vi "Start Measurements.vi"(6 "Reply to":refnum<class "Result Reply Msg.lvclass">, 7 "Objects enqueuers":refnum<class "Message Enqueuer.lvclass">[](array[class]), 8 "error in (no error)":errorcluster, 10 "Objects":string[](array[string]), 11 "Monitor Controller in":refnum<class "Monitor Controller.lvclass">) -> (0 "error out":errorcluster, 3 "Monitor Controller out":refnum<class "Monitor Controller.lvclass">)   [LabVIEW 2016, in "Monitor Controller.lvclass"]
uses:
  Monitor Controller.lvclass
  C:/github/LabActor/Worker/Worker.lvclass
  C:/github/LabActor/Controllers/Process Controller/Process Controller.lvclass
  Template Module Messages/Result Reply Msg/Result Reply Msg.lvclass
  <vilib>/ActorFramework/Message Enqueuer/Message Enqueuer.lvclass
  Worker/Worker.lvclass/Worker.ctl
  Monitor Controller.lvclass/Monitor Controller.ctl
  Process Controller/Process Controller.lvclass/Process Controller.ctl
  Worker/Write Cycle period.vi
  Process Controller/Write Repeat times.vi
  Process Controller/Write Timestamp data points.vi
  Template Module/Read State.vi
  Read Monitor controller configuration.vi
  Process Controller/Process Controller.lvclass
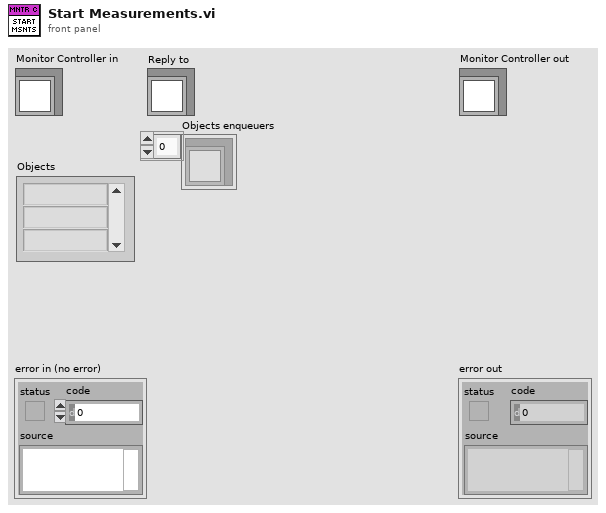
[diagram p1: front panel]
types:
  T1 = typedef "Worker State.ctl" = enum16{"Idle", "Starting", "Working", "Stopping"}
  T2 = typedef "Monitor Controller Configuration.ctl" = cluster{"Update period":dbl, "Repeat times":i32, "Open plot":bool, "File defragment period":dbl, "Timestamp data points":bool, "Re-plot rate limit":dbl}
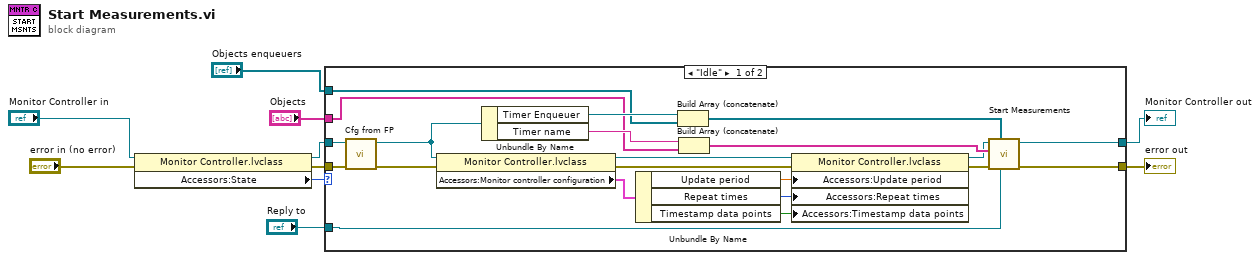
[diagram p0: block diagram]
diagram:
  n1 = property class="Monitor Controller.lvclass"(reference="Monitor Controller in", error in="error in (no error)") -> (reference out=w5:refnum<class "Monitor Controller.lvclass">, error out=w3:errorcluster, "Accessors:State"=w1:T1)
  n2 = case shown="\"Idle\"" w1 {
    tunnel: "Reply to" -> [w31 _]
    tunnel: "Objects enqueuers" -> [w29 _]
    tunnel: "Objects" -> [w27 _]
    tunnel: [w23 w32] -> w6
    tunnel: w5 -> [w15 w33]
    tunnel: w3 -> [w14 w32]
    tunnel: [w24 w33] -> w2
    frame "Idle" {
      n3 = call-dynamic "Cfg from FP.vi"("error in (no error)"=w14, "Measure Object in"=w15) -> ("error out"=w13:errorcluster, "Measure Object out"=w12:refnum<class "Monitor Controller.lvclass">)  [unwired: 8 in]
      n4 = property class="Monitor Controller.lvclass"(reference=w12, error in=w13) -> (reference out=w21:refnum<class "Monitor Controller.lvclass">, error out=w17:errorcluster, "Accessors:Monitor controller configuration"=w20:T2)
      n5 = Unbundle By Name(w12) -> ("Timer Enqueuer"=w30:refnum<class "Message Enqueuer.lvclass">, "Timer name"=w28:string)
      n6 = Unbundle By Name(w20) -> ("Update period"=w19:dbl, "Repeat times"=w16:i32, "Timestamp data points"=w11:bool)
      n7 = Build Array (concatenate)(w30, w29) -> (w26:refnum<class "Message Enqueuer.lvclass">[])
      n8 = Build Array (concatenate)(w28, w27) -> (w25:string[])
      n9 = property class="Monitor Controller.lvclass"(reference=w21, error in=w17, "Accessors:Update period"=w19, "Accessors:Repeat times"=w16, "Accessors:Timestamp data points"=w11) -> (reference out=w22:refnum<class "Monitor Controller.lvclass">, error out=w18:errorcluster)
      n10 = call-parent "Start Measurements.vi"("Reply to"=w31, "Objects enqueuers"=w26, "error in (no error)"=w18, "Objects"=w25, "Measure Controller in"=w22) -> ("error out"=w23:errorcluster, "Measure Controller out"=w24:refnum<class "Monitor Controller.lvclass">)  [unwired: 5 in]
    }
    frame "Working", Default {
    }
  }
  "error out" <- w6
  "Monitor Controller out" <- w2
